vi "Create New Azure Container.vi"() -> ()   [LabVIEW 2015]
doc: "Demonstrates the use of the <b>Create Container</b> VI in the NI Cloud Toolkit for Azure."
uses:
  Core/Azure Credentials.ctl
  Blob Storage/NI_Azure_Blob.lvlib
  Core/Session/Session.lvclass
  Core/NI_Azure_Core.lvlib
panel:
  in  "Access Key":string
  in  "Storage Account Name":string
  in  "Container Name":string
  # "Overview: Demonstrates how to create a new container for the Azure Blob Service.\nRequirements: NI Cloud Toolkit for Azure and a registered Microsoft Azure account\nInstructions:\n1. Specify the Storage Account Name and Access Key for your Azure account. You can create an account at https://azure.microsoft.com.\n2. Specify Container Name for the container you want to create.\n3. Run the VI. Verify in the Microsoft Azure console that the specified container was created."
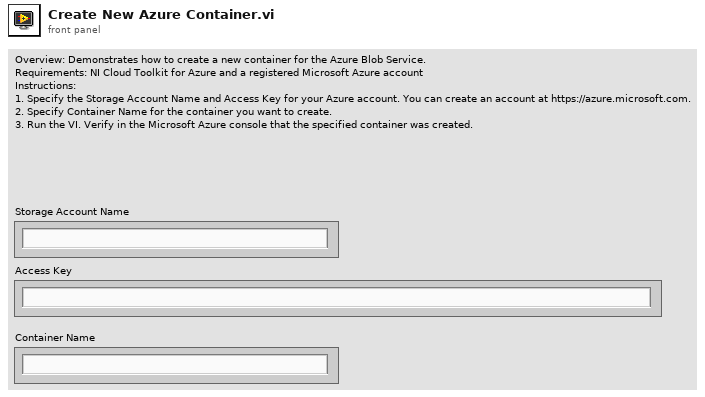
[diagram p1: front panel]
types:
  T1 = typedef "NI_Azure_Core.lvlib/Azure Credentials.ctl" = cluster{"Storage Account Name":string, "Access Key":string}
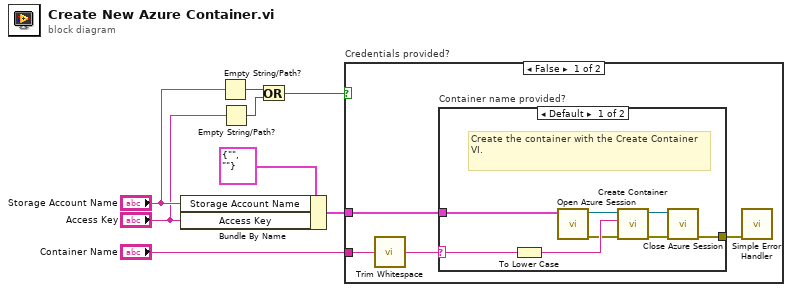
[diagram p0: block diagram]
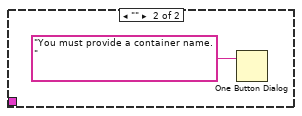
[diagram p2: hidden frame]
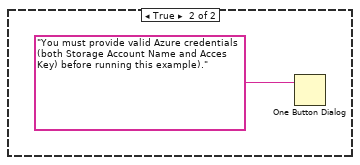
[diagram p3: hidden frame]
diagram:
  n1 = Bundle By Name(cluster=T1 {"Storage Account Name"="", "Access Key"=""} ("Credentials"), "Storage Account Name"="Storage Account Name", "Access Key"="Access Key") -> (w8:T1)
  n2 = Empty String/Path?(string/path="Storage Account Name") -> (empty?=w7:bool)
  n3 = Empty String/Path?(string/path="Access Key") -> (empty?=w5:bool)
  n4 = Or(x=w7, y=w5) -> (x .or. y?=w6:bool)
  n5 = case "Credentials provided?" shown="False" w6 {
    tunnel: w8 -> [w12 _]
    tunnel: "Container Name" -> [w10 _]
    frame False {
      n6 = call <vilib>:"Trim Whitespace.vi"("string"=w10) -> ("trimmed string"=w9:string)  [unwired: 1 in]
      n7 = case "Container name provided?" shown="Default" w9 {
        selector: w9 -> [w20 _]
        tunnel: w12 -> [w13 _]
        tunnel: [w15 _] -> w11
        frame Default {
          # "Create the container with the Create Container VI."
          n8 = To Lower Case(string=w20) -> (all lower case string=w18:string)
          n9 = call "Open Azure Session.vi"("Credentials"=w13) -> ("error out"=w16:errorcluster, "Azure Session"=w17:refnum<class "Session.lvclass">)  [unwired: 9 in]
          n10 = call "Create Container.vi"("error in (no error)"=w16, "Container"=w18, "Azure Session in"=w17) -> ("error out"=w19:errorcluster, "Azure Session out"=w14:refnum<class "Session.lvclass">)  [unwired: 7 in]
          n11 = call "Close Azure Session.vi"("error in (no error)"=w19, "Azure Session"=w14) -> ("error out"=w15:errorcluster)  [unwired: 9 in]
        }
        frame "" {
          n12 = One Button Dialog(message="You must provide a container name.") -> ()  [unwired: 1 in, 1 out]
        }
      }
      n13 = call <vilib>:"Simple Error Handler.vi"("error in (no error)"=w11) -> ()  [unwired: 4 in, 5 out]
    }
    frame True {
      n14 = One Button Dialog(message="You must provide valid Azure credentials (both Storage Account Name and Acces Key) before running this example).") -> ()  [unwired: 1 in, 1 out]
    }
  }
